vi "main.vi"() -> ()   [LabVIEW 2020]
panel:
  in  "Boolean 2":bool
  out "Boolean":bool
  out "Waveform Chart":dbl(graph)
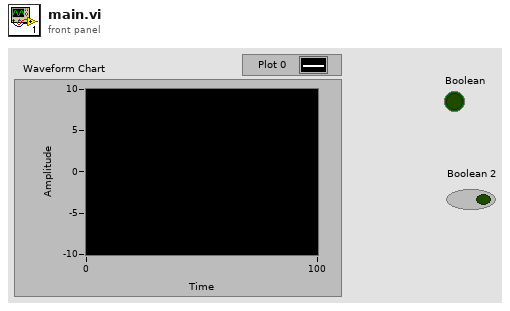
[diagram p1: front panel]
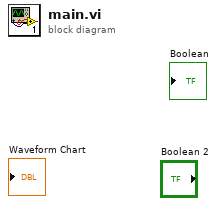
[diagram p0: block diagram]
diagram:
